vi "Write FP Control.vi"(8 "error in (no error)":errorcluster, 9 "Control Value":variant, 10 "Control Name":string="Parameters", 11 "Mag Lab Root in":refnum<class "Mag Lab Root.lvclass">) -> (0 "error out":errorcluster, 3 "Mag Lab Root out":refnum<class "Mag Lab Root.lvclass">)   [LabVIEW 2015, in "Mag Lab Root.lvclass"]
uses:
  Mag Lab Root.lvclass
  Mag Lab Root.lvclass/Mag Lab Root.ctl
  Read Front Panel ref.vi
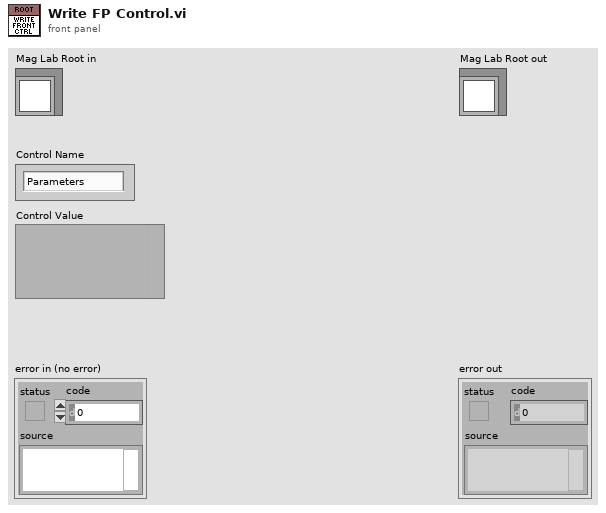
[diagram p1: front panel]
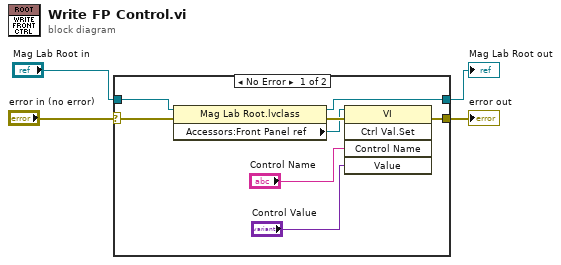
[diagram p0: block diagram]
diagram:
  n1 = case shown="No Error" "error in (no error)" {
    selector: "error in (no error)" -> [w6 w14]
    tunnel: [w7 w14] -> w3
    tunnel: [w9 w13] -> w1
    tunnel: "Mag Lab Root in" -> [w10 w13]
    frame No Error {
      n2 = property class="Mag Lab Root.lvclass"(reference=w10, error in=w6) -> (reference out=w9:refnum<class "Mag Lab Root.lvclass">, error out=w12:errorcluster, "Accessors:Front Panel ref"=w11:refnum<vi>)
      n3 = invoke class="VI" method="Ctrl Val.Set"(reference=w11, error in=w12, "Control Name"="Control Name", "Value"="Control Value") -> (error out=w7:errorcluster)  [unwired: 1 in, 4 out]
    }
    frame Error {
    }
  }
  "error out" <- w3
  "Mag Lab Root out" <- w1
